vi "Contex Menu Selection.vi"(8 "error in (no error)":errorcluster, 10 "MenuItem":string, 11 "HIJ Vision Display in":refnum<class "HIJ Vision Display.lvclass">) -> (0 "error out":errorcluster, 3 "HIJ Vision Display out":refnum<class "HIJ Vision Display.lvclass">)   [LabVIEW 2014, in "HIJ Vision Display.lvlib" / "HIJ Vision Display.lvclass"]
uses:
  HIJ Vision Display.lvclass
  HIJ Vision Display.lvclass/HIJ Vision Display.ctl
  Read Display ref.vi
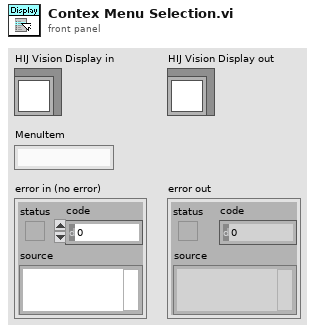
[diagram p1: front panel]
types:
  T1 = typedef "ROI Descriptor" = cluster{"Global Rectangle":i32[], "Contours":cluster{"ID":enum32{"External", "Internal"}, "Type":u32, "Coordinates":i32[]}[]}
  T2 = cluster{"Global Rectangle":i32[], "Contours":cluster{"Contour Type":u32, "ROI Type":u32, "Points":i32[]}[]}
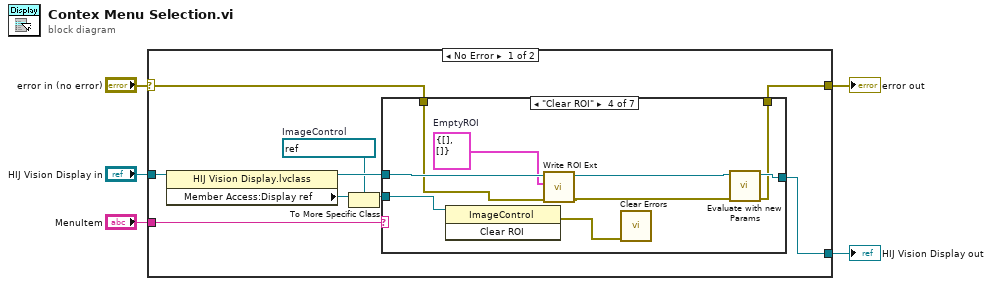
[diagram p0: block diagram]
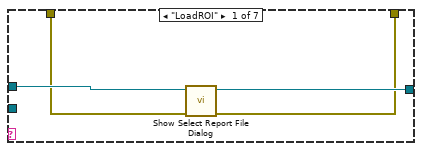
[diagram p2: hidden frame]
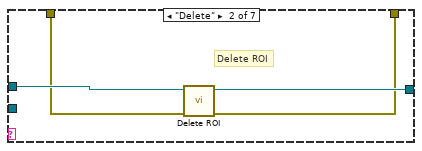
[diagram p3: hidden frame]
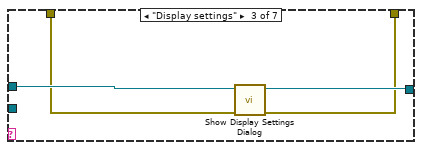
[diagram p4: hidden frame]
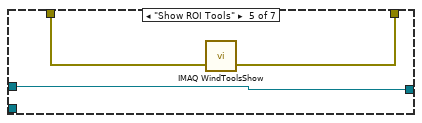
[diagram p5: hidden frame]
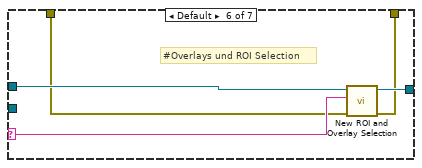
[diagram p6: hidden frame]
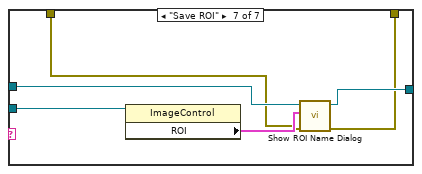
[diagram p7: hidden frame]
diagram:
  n1 = case shown="No Error" "error in (no error)" {
    selector: "error in (no error)" -> [w8 w51]
    tunnel: [w7 w51] -> w4
    tunnel: [w9 w50] -> w2
    tunnel: "HIJ Vision Display in" -> [w13 w50]
    tunnel: "MenuItem" -> [w14 _]
    frame No Error {
      w6 = refnum<vi> refnum  # ImageControl
      n2 = property class="HIJ Vision Display.lvclass"(reference=w13) -> (reference out=w10:refnum<class "HIJ Vision Display.lvclass">, "Member Access:Display ref"=w12:refnum<vi>)  [unwired: 1 in, 1 out]
      n3 = To More Specific Class(target class=w6, reference=w12) -> (specific class reference=w11:refnum<vi>)  [unwired: 1 in, 1 out]
      n4 = case shown="\"Clear ROI\"" w14 {
        selector: w14 -> [_ _ _ _ _ w41 _]
        tunnel: w11 -> [_ _ _ w34 _ _ w49]
        tunnel: w10 -> [w18 w22 w26 w33 w38 w43 w48]
        tunnel: [w17 w20 w25 w32 w38 w42 w47] -> w9
        tunnel: w8 -> [w16 w21 w24 w28 w37 w40 w45]
        tunnel: [w15 w19 w23 w31 w36 w39 w44] -> w7
        frame "LoadROI" {
          n5 = call "Show Select Report File Dialog.vi"("error in (no error)"=w16, "IMAQ Display in"=w18) -> ("error out"=w15:errorcluster, "IMAQ Display out"=w17:refnum<class "HIJ Vision Display.lvclass">)  [unwired: 8 in]
        }
        frame "Delete" {
          # "Delete ROI"
          n6 = call "Delete ROI.vi"("error in (no error)"=w21, "IMAQ Display in"=w22) -> ("error out"=w19:errorcluster, "IMAQ Display out"=w20:refnum<class "HIJ Vision Display.lvclass">)  [unwired: 8 in]
        }
        frame "Display settings" {
          n7 = call "Show Display Settings Dialog.vi"("error in (no error)"=w24, "IMAQ Display in"=w26) -> ("error out"=w23:errorcluster, "IMAQ Display out"=w25:refnum<class "HIJ Vision Display.lvclass">)  [unwired: 8 in]
        }
        frame "Clear ROI" {
          w29 = T1 {"Global Rectangle"=[], "Contours"=[]}  # EmptyROI
          n8 = invoke on="Invoke Node" class="ImageControl" method="Clear ROI"(reference=w34) -> (error out=w35:errorcluster)  [unwired: 2 in, 2 out]
          n9 = call "Write ROI Ext.vi"("error in (no error)"=w28, "ROI Descriptor"=w29, "IMAQ Display in"=w33) -> ("error out"=w27:errorcluster, "IMAQ Display out"=w30:refnum<class "HIJ Vision Display.lvclass">)  [unwired: 7 in]
          n10 = call <vilib>:"Clear Errors.vi"("error in (no error)"=w35) -> ()  [unwired: 5 in, 2 out]
          n11 = call-dynamic "Evaluate with new Params.vi"("error in (no error)"=w27, "HIJ Vision Display in"=w30) -> ("error out"=w31:errorcluster, "HIJ Vision Display out"=w32:refnum<class "HIJ Vision Display.lvclass">)  [unwired: 8 in]
        }
        frame "Show ROI Tools" {
          n12 = call "IMAQ WindToolsShow"("error in (no error)"=w37) -> ("error out"=w36:errorcluster)  [unwired: 4 in, 1 out]
        }
        frame Default {
          # "#Overlays und ROI Selection"
          n13 = call-dynamic "New ROI and Overlay Selection.vi"("error in (no error)"=w40, "ItemTag"=w41, "IMAQ Display in"=w43) -> ("error out"=w39:errorcluster, "IMAQ Display out"=w42:refnum<class "HIJ Vision Display.lvclass">)  [unwired: 7 in]
        }
        frame "Save ROI" {
          n14 = property on="Property Node" class="ImageControl"(reference=w49) -> ("ROI"=w46:T2)  [unwired: 1 in, 2 out]
          n15 = call-dynamic "Show ROI Name Dialog.vi"("error in (no error)"=w45, "ROI Descriptor"=w46, "IMAQ Display in"=w48) -> ("error out"=w44:errorcluster, "IMAQ Display out"=w47:refnum<class "HIJ Vision Display.lvclass">)  [unwired: 7 in]
        }
      }
    }
    frame Error {
    }
  }
  "error out" <- w4
  "HIJ Vision Display out" <- w2
